vi "Configuration Resistance.vi"(0 "VISA resource name":refnum<visa-resource-name>, 1 "High/Low (1:High)":u8(slide)=1 scale=0.0..1.0, 2 "Rise (3.2)":sgl=3.2 min=0 step=3.2 format="%.2f", 3 "Fall (3.2)":sgl=3.2 min=0 step=3.2 format="%.2f", 5 "Channel 1-8 (0:Ch1)":u8(ring) items=["Channel 1", "Channel 2", "Channel 3", "Channel 4", "Channel 5", "Channel 6", "Channel 7", "Channel 8 "], 7 "Resistance Level (7.5 Ohm)":sgl=7.5 min=0 format="%^.4e", 11 "error in (no error)":errorcluster) -> (4 "VISA resource name out":refnum<visa-resource-name>, 15 "error out":errorcluster)   [LabVIEW 2015, in "Chroma ATE 6310.lvlib"]
doc: "This function sets the constant resistance mode.\n\nIn CR mode, the Load will sink a current linearly propotional to the input voltage in accordance with the programmed resistance."
uses:
  <instrlib>/Chroma ATE 6310/Chroma ATE 6310.lvlib
panel:
  # "Slew Rate\n(mA/uS)"
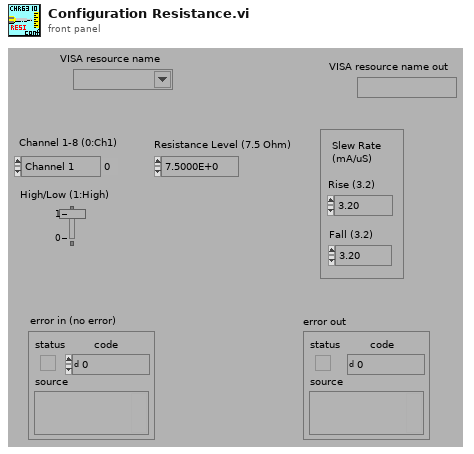
[diagram p1: front panel]
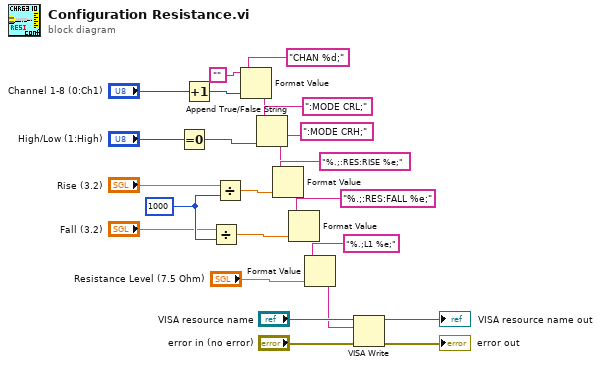
[diagram p0: block diagram]
diagram:
  w8 = 1000
  n1 = Equal To 0?(x="High/Low (1:High)") -> (x = 0?=w11:bool)
  n2 = Increment(x="Channel 1-8 (0:Ch1)") -> (x+1=w23:u8)
  n3 = Divide(x="Fall (3.2)", y=w8) -> (x/y=w9:sgl)
  n4 = Divide(x="Rise (3.2)", y=w8) -> (x/y=w10:sgl)
  n5 = Format Value(string ("")="", format string="CHAN %d;", value (0)=w23) -> (output string=w13:string)
  n6 = Append True/False String(1:w11, 2:":MODE CRH;", 3:":MODE CRL;", 4:w13) -> (0:w12:string)
  n7 = Format Value(string ("")=w12, format string="%.;:RES:RISE %e;", value (0)=w10) -> (output string=w20:string)
  n8 = Format Value(string ("")=w20, format string="%.;:RES:FALL %e;", value (0)=w9) -> (output string=w18:string)
  n9 = Format Value(string ("")=w18, format string="%.;L1 %e;", value (0)="Resistance Level (7.5 Ohm)") -> (output string=w1:string)
  n10 = VISA Write(VISA resource name="VISA resource name", write buffer=w1, error in (no error)="error in (no error)") -> (VISA resource name out=→"VISA resource name out":refnum<visa-resource-name>, error out=→"error out":errorcluster)  [unwired: 1 out]
